vi "Histogram Main.vi"() -> ()   [LabVIEW 2015]
uses:
  Consumer Message.ctl
  <vilib>/ErrorRing/Error Ring.xnode
panel:
  in  "bins":i32=20
  in  "signal":u16(ring) items=["uniform white", "uniform+uniform", "Gaussian white", "sine", "square"]
  out "Consumer Shutdown?":bool
  out "Backlog":u8(slide) scale=0.0..100.0
  in  "High Priority Message":bool
  in  "Normal Priority Message":bool
  in  "Stop":bool
  # "Number of enqueued messages waiting to be processed"
  # "Current data being processed in consumer loop"
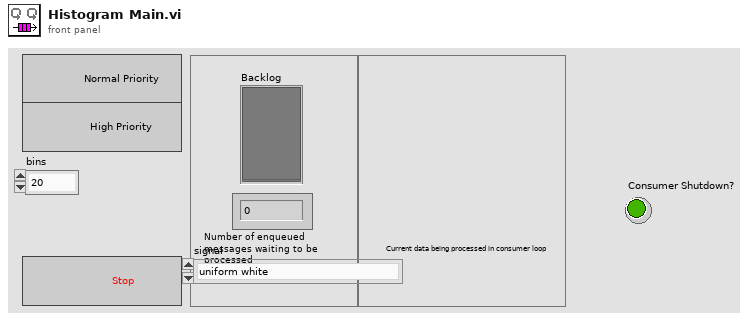
[diagram p1: front panel]
types:
  T1 = typedef "Consumer Message.ctl" = cluster{"Consumer State":string, "Boolean Data":bool, "Numeric Data":i32, "Signal":dbl[], "Error":errorcluster}
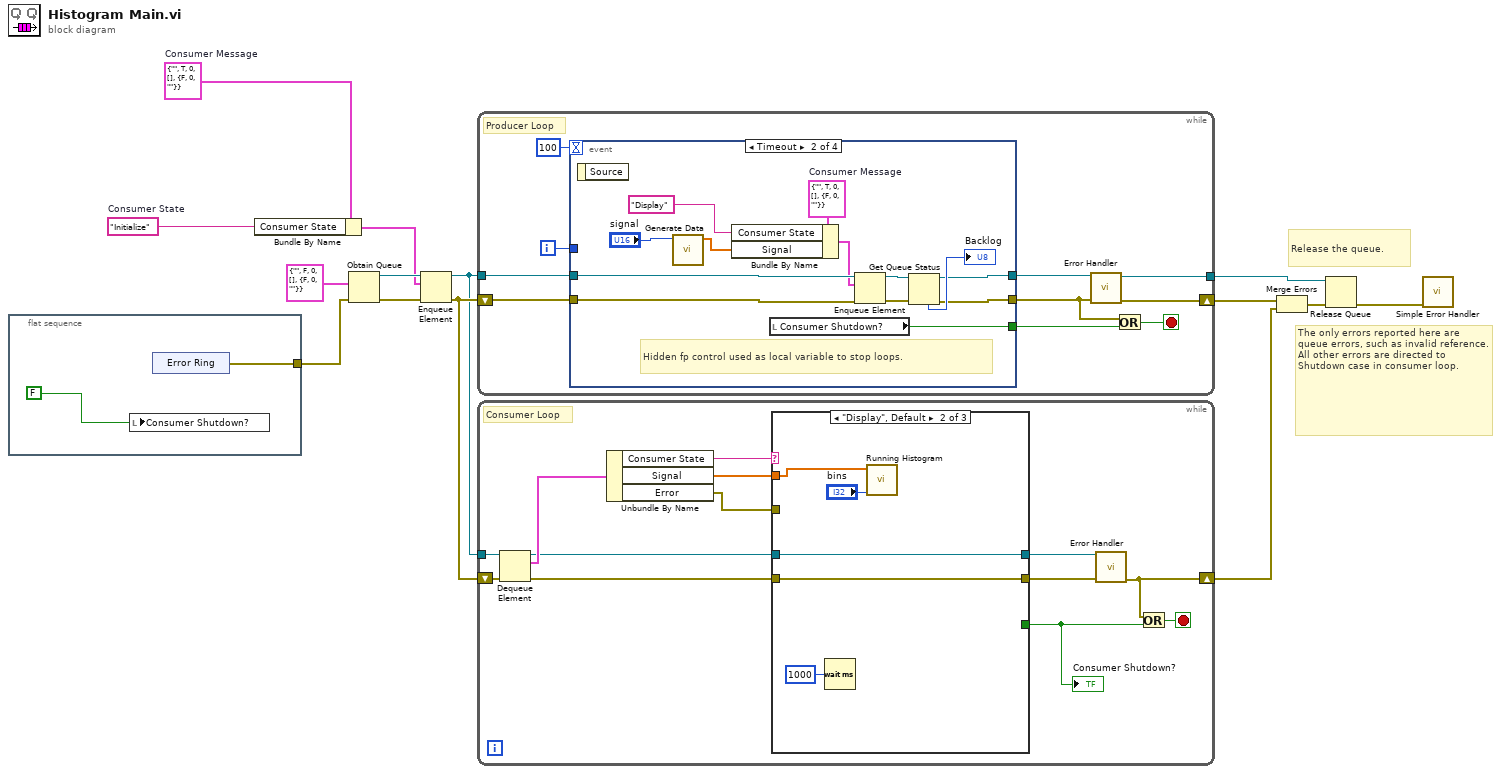
[diagram p0: block diagram]
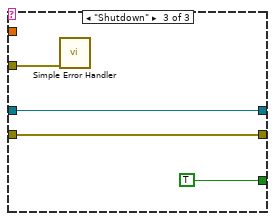
[diagram p3: hidden frame]
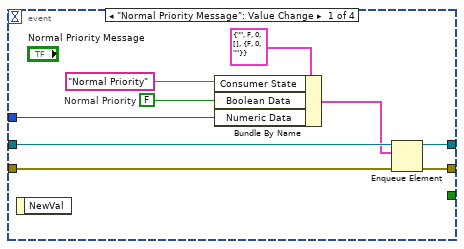
[diagram p4: hidden frame]
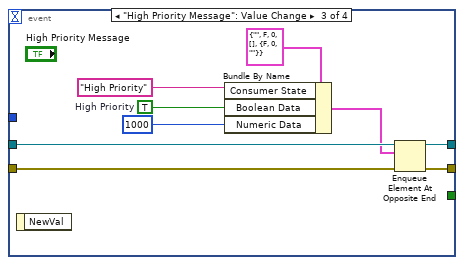
[diagram p5: hidden frame]
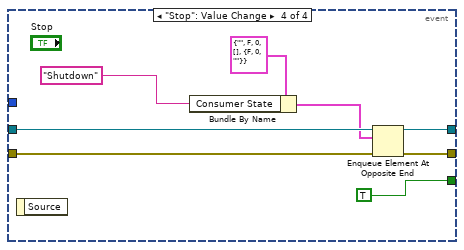
[diagram p6: hidden frame]
diagram:
  w6 = "Initialize"  # Consumer State
  w8 = T1 {"Consumer State"="", "Boolean Data"=TRUE, "Numeric Data"=0, "Signal"=[], "Error"={"status"=FALSE, "code"=0, "source"=""}}  # Consumer Message
  # "Release the queue."
  # "The only errors reported here are queue errors, such as invalid reference.  All other errors are directed to Shutdown case in consumer loop."
  n1 = flat-sequence {
    tunnel: [w15] -> w9
    frame #0 {
      n2 = local write "Consumer Shutdown?"(FALSE ("Stop Loops (local)")) -> ()
      n3 = xnode "Error Ring"() -> ("error out"=w15:errorcluster)
    }
  }
  n4 = Bundle By Name(cluster=w8, "Consumer State"=w6) -> (w7:T1)
  n5 = Obtain Queue(element data type=T1 {"Consumer State"="", "Boolean Data"=FALSE, "Numeric Data"=0, "Signal"=[], "Error"={"status"=FALSE, "code"=0, "source"=""}}, error in (no error)=w9) -> (queue out=w11:refnum<queue>, error out=w14:errorcluster)  [unwired: 3 in, 1 out]
  n6 = Enqueue Element(queue=w11, element=w7, error in (no error)=w14) -> (queue out=w10:refnum<queue>, error out=w12:errorcluster)  [unwired: 1 in, 1 out]
  n7 = while {
    tunnel: w10 -> [w27]
    shift-right: [w19] -> w5
    shift-left: w12 -> [w26]
    tunnel: [w18] -> w1
    i -> [w25]
    stop <- w21 stop-if-true
    # "Producer Loop"
    n8 = event shown="[1] Timeout" {
      selector: _ -> [_ _ _ _]
      dyn-events: _ -> [_ _ _ _]
      timeout: 100 -> [_ _ _ _]
      tunnel: w27 -> [w36 w47 w57 w66]
      tunnel: w26 -> [w34 w39 w56 w64]
      tunnel: [w35 w46 w58 w63] -> w20
      tunnel: [_ w49 _ TRUE] -> w22
      tunnel: w25 -> [w33 _ _ _]
      tunnel: [w29 w45 w52 w62] -> w24
      event "Normal Priority Message": Value Change {
        w30 = FALSE  # Normal Priority
        n9 = event-data() -> ()  [unwired: 1 in, 1 out]
        n10 = Bundle By Name(cluster=T1 {"Consumer State"="", "Boolean Data"=FALSE, "Numeric Data"=0, "Signal"=[], "Error"={"status"=FALSE, "code"=0, "source"=""}}, "Consumer State"="Normal Priority" ("String Data"), "Boolean Data"=w30, "Numeric Data"=w33) -> (w32:T1)
        n11 = Enqueue Element(queue=w36, element=w32, error in (no error)=w34) -> (queue out=w29:refnum<queue>, error out=w35:errorcluster)  [unwired: 1 in, 1 out]
      }
      event Timeout {
        w44 = T1 {"Consumer State"="", "Boolean Data"=TRUE, "Numeric Data"=0, "Signal"=[], "Error"={"status"=FALSE, "code"=0, "source"=""}}  # Consumer Message
        # "Hidden fp control used as local variable to stop loops."
        n12 = event-data() -> ()  [unwired: 1 in, 1 out]
        n13 = call "Generate Data.vi"("signal"="signal") -> ("Y"=w43:dbl[])  [unwired: 9 in, 1 out]
        n14 = Bundle By Name(cluster=w44, "Consumer State"="Display", "Signal"=w43) -> (w37:T1)
        n15 = local read "Consumer Shutdown?"() -> (w49:bool)
        n16 = Enqueue Element(queue=w47, element=w37, error in (no error)=w39) -> (queue out=w40:refnum<queue>, error out=w38:errorcluster)  [unwired: 1 in, 1 out]
        n17 = Get Queue Status(queue=w40, error in (no error)=w38) -> (queue out=w45:refnum<queue>, error out=w46:errorcluster, # elements in queue=→"Backlog":i32)  [unwired: 1 in, 5 out]
      }
      event "High Priority Message": Value Change {
        w51 = TRUE  # High Priority
        n18 = event-data() -> ()  [unwired: 1 in, 1 out]
        n19 = Bundle By Name(cluster=T1 {"Consumer State"="", "Boolean Data"=FALSE, "Numeric Data"=0, "Signal"=[], "Error"={"status"=FALSE, "code"=0, "source"=""}}, "Consumer State"="High Priority" ("String Data"), "Boolean Data"=w51, "Numeric Data"=1000) -> (w54:T1)
        n20 = Enqueue Element At Opposite End(queue=w57, element=w54, error in (no error)=w56) -> (queue out=w52:refnum<queue>, error out=w58:errorcluster)  [unwired: 1 in, 1 out]
      }
      event "Stop": Value Change {
        n21 = event-data() -> ()  [unwired: 1 in, 1 out]
        n22 = Bundle By Name(cluster=T1 {"Consumer State"="", "Boolean Data"=FALSE, "Numeric Data"=0, "Signal"=[], "Error"={"status"=FALSE, "code"=0, "source"=""}}, "Consumer State"="Shutdown") -> (w59:T1)
        n23 = Enqueue Element At Opposite End(queue=w66, element=w59, error in (no error)=w64) -> (queue out=w62:refnum<queue>, error out=w63:errorcluster)  [unwired: 1 in, 1 out]
      }
    }
    n24 = call "Error Handler.vi"("error in"=w20, "queue in"=w24) -> ("error out"=w19:errorcluster, "queue out"=w18:refnum<queue>)  [unwired: 8 in]
    n25 = Or(x=w20, y=w22) -> (x .or. y?=w21:bool)
  }
  n26 = while {
    tunnel: w10 -> [w79]
    shift-right: [w69] -> w4
    shift-left: w12 -> [w78]
    stop <- w70 stop-if-true
    # "Consumer Loop"
    n27 = Dequeue Element(queue=w79, error in (no error)=w78) -> (queue out=w68:refnum<queue>, element=w77:T1, error out=w67:errorcluster)  [unwired: 1 in, 1 out]
    n28 = Unbundle By Name(w77) -> ("Consumer State"=w76:string, "Signal"=w75:dbl[], "Error"=w72:errorcluster)
    n29 = case shown="\"Display\", Default" w76 {
      tunnel: [_ _ TRUE] -> w71
      tunnel: w67 -> [w80 w84 w87]
      tunnel: [w80 w84 w87] -> w74
      tunnel: w75 -> [_ w83 _]
      tunnel: w68 -> [w81 w86 w88]
      tunnel: [w81 w86 w88] -> w73
      tunnel: w72 -> [_ _ w89]
      frame "Initialize" {
      }
      frame "Display", Default {
        n30 = Wait (ms)(milliseconds to wait=u32 1000) -> ()  [unwired: 1 out]
        n31 = call "Running Histogram.vi"("bins"="bins", "input data"=w83) -> ()  [unwired: 6 in, 4 out]
      }
      frame "Shutdown" {
        n32 = call <vilib>:"Simple Error Handler.vi"("error in (no error)"=w89) -> ()  [unwired: 4 in, 5 out]
      }
    }
    "Consumer Shutdown?" <- w71
    n33 = call "Error Handler.vi"("error in"=w74, "queue in"=w73) -> ("error out"=w69:errorcluster)  [unwired: 8 in, 1 out]
    n34 = Or(x=w69, y=w71) -> (x .or. y?=w70:bool)
  }
  n35 = Merge Errors(w5, w4) -> (w3:errorcluster)
  n36 = Release Queue(queue=w1, error in (no error)=w3) -> (error out=w2:errorcluster)  [unwired: 1 in, 2 out]
  n37 = call <vilib>:"Simple Error Handler.vi"("error in (no error)"=w2) -> ()  [unwired: 4 in, 5 out]
